vi "Wire N Reserve Session Inputs.vi"(0 "SubVI in":refnum<vi>, 5 "vi reference":refnum<vi>, 7 "Build Array":refnum<vi>, 11 "error in (no error)":errorcluster) -> (15 "error out":errorcluster)   [LabVIEW 2021, in "Converter.lvlib"]
uses:
  Converter.lvlib
  Converter Reusables/Converter Reusables.lvlib
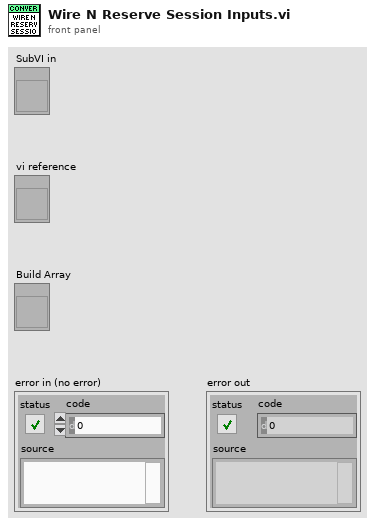
[diagram p1: front panel]
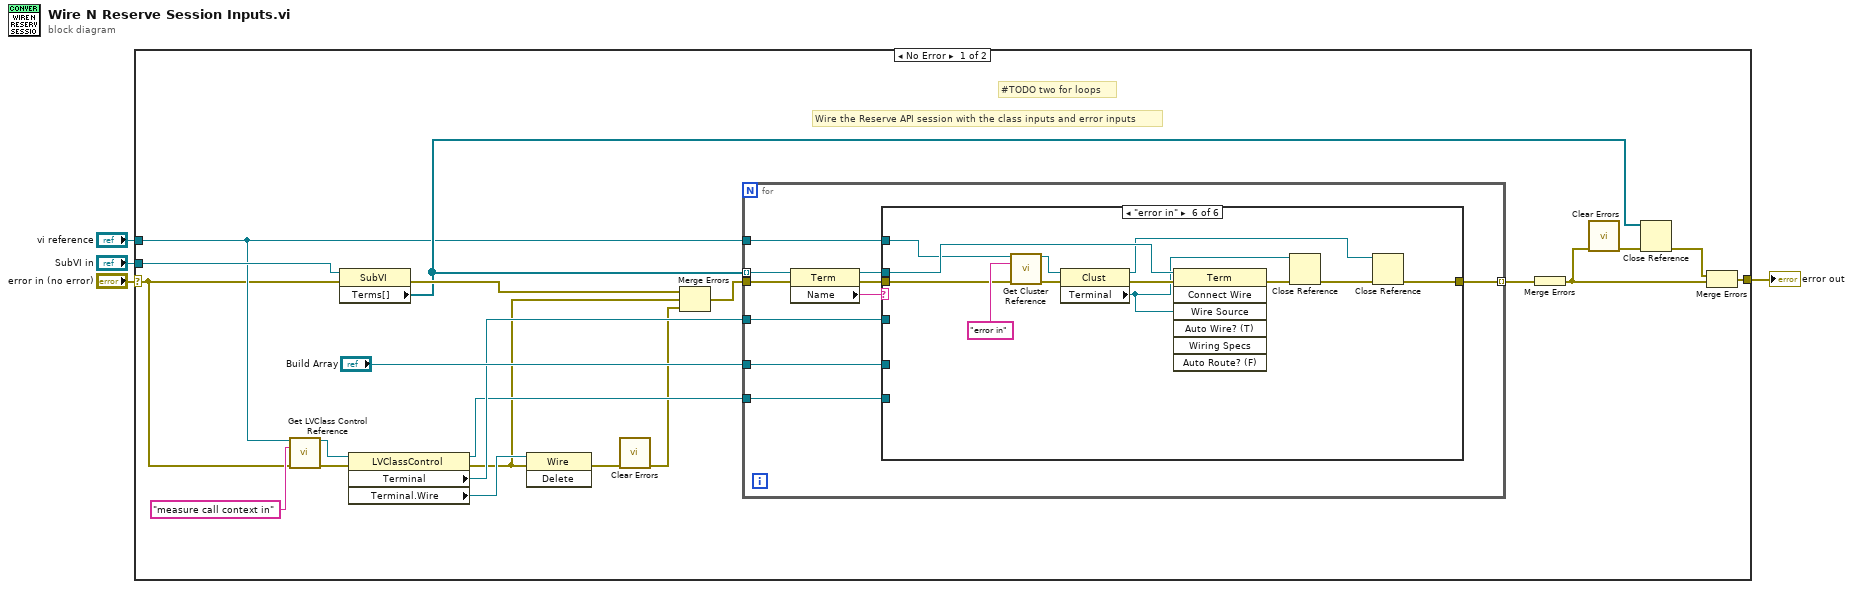
[diagram p0: block diagram]
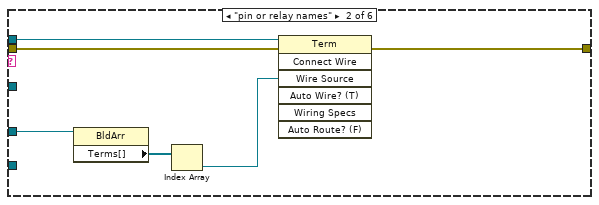
[diagram p3: hidden frame]
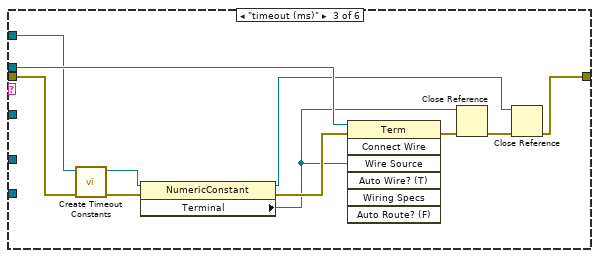
[diagram p4: hidden frame]
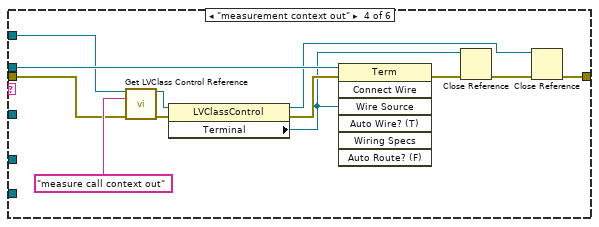
[diagram p5: hidden frame]
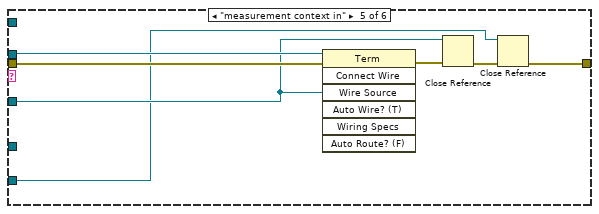
[diagram p6: hidden frame]
diagram:
  n1 = case shown="No Error" "error in (no error)" {
    selector: "error in (no error)" -> [w9 w85]
    tunnel: "SubVI in" -> [w23 _]
    tunnel: [w19 w85] -> w3
    tunnel: "vi reference" -> [w14 _]
    frame No Error {
      # "Wire the Reserve API session with the class inputs and error inputs"
      # "#TODO two for loops"
      n2 = call "Get LVClass Control Reference.vi"("VI in"=w14, "name/order"="measure call context in", "error in (no error)"=w9) -> ("Cluster out"=w11:refnum<vi>, "error out"=w15:errorcluster)  [unwired: 11 in]
      n3 = property class="SubVI"(reference=w23, error in=w9) -> (error out=w24:errorcluster, "Terms[]"=w22:refnum<vi>[])  [unwired: 1 out]
      n4 = property class="LVClassControl"(reference=w11, error in=w15) -> (reference out=w10:refnum<vi>, error out=w7:errorcluster, "Terminal"=w12:refnum<vi>, "Terminal.Wire"=w16:refnum<vi>)
      n5 = invoke class="Wire" method="Delete"(reference=w16, error in=w7) -> (error out=w6:errorcluster)  [unwired: 1 in, 2 out]
      n6 = call <vilib>:"Clear Errors.vi"("error in (no error)"=w6) -> ("error out"=w5:errorcluster)  [unwired: 5 in, 1 out]
      n7 = Merge Errors(w24, w7, w5) -> (w8:errorcluster)
      n8 = for {
        tunnel: w22 -> [w35] mode=indexing
        tunnel: w8 -> [w34]
        tunnel: [w30] -> w25 mode=indexing
        tunnel: w14 -> [w29]
        tunnel: "Build Array" -> [w28]
        tunnel: w12 -> [w27]
        tunnel: w10 -> [w26]
        n9 = property class="Term"(reference=w35, error in=w34) -> (reference out=w31:refnum<vi>, error out=w32:errorcluster, "Name"=w33:string)
        n10 = case shown="\"error in\"" w33 {
          tunnel: w32 -> [w36 w41 w43 w61 w71 w80]
          tunnel: w31 -> [_ w42 w53 w65 w72 w84]
          tunnel: [w36 w40 w50 w56 w69 w76] -> w30
          tunnel: w29 -> [_ _ w49 w55 _ w83]
          tunnel: w28 -> [_ w39 _ _ _ _]
          tunnel: w27 -> [_ _ _ _ w67 _]
          tunnel: w26 -> [_ _ _ _ w66 _]
          frame Default {
          }
          frame "pin or relay names" {
            n11 = property class="BldArr"(reference=w39) -> ("Terms[]"=w38:refnum<vi>[])  [unwired: 1 in, 2 out]
            n12 = Index Array(array=w38) -> (element=w37:refnum<vi>)  [unwired: 1 in]
            n13 = invoke class="Term" method="Connect Wire"(reference=w42, error in=w41, "Wire Source"=w37) -> (error out=w40:errorcluster)  [unwired: 4 in, 6 out]
          }
          frame "timeout (ms)" {
            n14 = call "Create Timeout Constants.vi"("error in (no error)"=w43, "VI in"=w49) -> ("error out"=w48:errorcluster, "NumericConstant out"=w45:refnum<vi>)  [unwired: 8 in]
            n15 = property class="NumericConstant"(reference=w45, error in=w48) -> (reference out=w44:refnum<vi>, error out=w47:errorcluster, "Terminal"=w46:refnum<vi>)
            n16 = invoke class="Term" method="Connect Wire"(reference=w53, error in=w47, "Wire Source"=w46) -> (error out=w52:errorcluster)  [unwired: 4 in, 6 out]
            n17 = Close Reference(reference=w46, error in (no error)=w52) -> (error out=w51:errorcluster)
            n18 = Close Reference(reference=w44, error in (no error)=w51) -> (error out=w50:errorcluster)
          }
          frame "measurement context out" {
            n19 = call "Get LVClass Control Reference.vi"("VI in"=w55, "name/order"="measure call context out", "error in (no error)"=w61) -> ("Cluster out"=w57:refnum<vi>, "error out"=w63:errorcluster)  [unwired: 11 in]
            n20 = property class="LVClassControl"(reference=w57, error in=w63) -> (reference out=w54:refnum<vi>, error out=w60:errorcluster, "Terminal"=w59:refnum<vi>)
            n21 = invoke class="Term" method="Connect Wire"(reference=w65, error in=w60, "Wire Source"=w59) -> (error out=w64:errorcluster)  [unwired: 4 in, 6 out]
            n22 = Close Reference(reference=w59, error in (no error)=w64) -> (error out=w58:errorcluster)
            n23 = Close Reference(reference=w54, error in (no error)=w58) -> (error out=w56:errorcluster)
          }
          frame "measurement context in" {
            n24 = invoke class="Term" method="Connect Wire"(reference=w72, error in=w71, "Wire Source"=w67) -> (error out=w68:errorcluster)  [unwired: 4 in, 6 out]
            n25 = Close Reference(reference=w67, error in (no error)=w68) -> (error out=w70:errorcluster)
            n26 = Close Reference(reference=w66, error in (no error)=w70) -> (error out=w69:errorcluster)
          }
          frame "error in" {
            n27 = call "Get Cluster Reference.vi"("VI in"=w83, "name/order"="error in", "error in (no error)"=w80) -> ("Cluster out"=w81:refnum<vi>, "error out"=w79:errorcluster)  [unwired: 11 in]
            n28 = property class="Clust"(reference=w81, error in=w79) -> (reference out=w77:refnum<vi>, error out=w78:errorcluster, "Terminal"=w73:refnum<vi>)
            n29 = invoke class="Term" method="Connect Wire"(reference=w84, error in=w78, "Wire Source"=w73) -> (error out=w74:errorcluster)  [unwired: 4 in, 6 out]
            n30 = Close Reference(reference=w73, error in (no error)=w74) -> (error out=w75:errorcluster)
            n31 = Close Reference(reference=w77, error in (no error)=w75) -> (error out=w76:errorcluster)
          }
        }
      }
      n32 = Merge Errors(w25) -> (w20:errorcluster)
      n33 = call <vilib>:"Clear Errors.vi"("error in (no error)"=w20) -> ("error out"=w17:errorcluster)  [unwired: 5 in, 1 out]
      n34 = Close Reference(reference=w22, error in (no error)=w17) -> (error out=w21:errorcluster)
      n35 = Merge Errors(w21, w20) -> (w19:errorcluster)
    }
    frame Error {
    }
  }
  "error out" <- w3
